vi "GainValue2Number.vi"(10 "GainValue":u64, 11 "Gain permitted values":u32[](array[numeric])=[0, 16, 32, 48, 64, 80, 96, 112, 128, 144, 160, 176, 192, 208, 224, 240, 256, 288, 320, 352, 384, 416, 448, 480, 512, 544, 576, 608, 640, 672, 704, 736, 768, 832, 896, 960, 1024, 1088, 1152, 1216, 1280, 1344, 1408, 1472, 1536, 1600, 1664, 1728]) -> (2 "Value out":u32, 3 "fractional index or x":dbl)   [LabVIEW 2015]
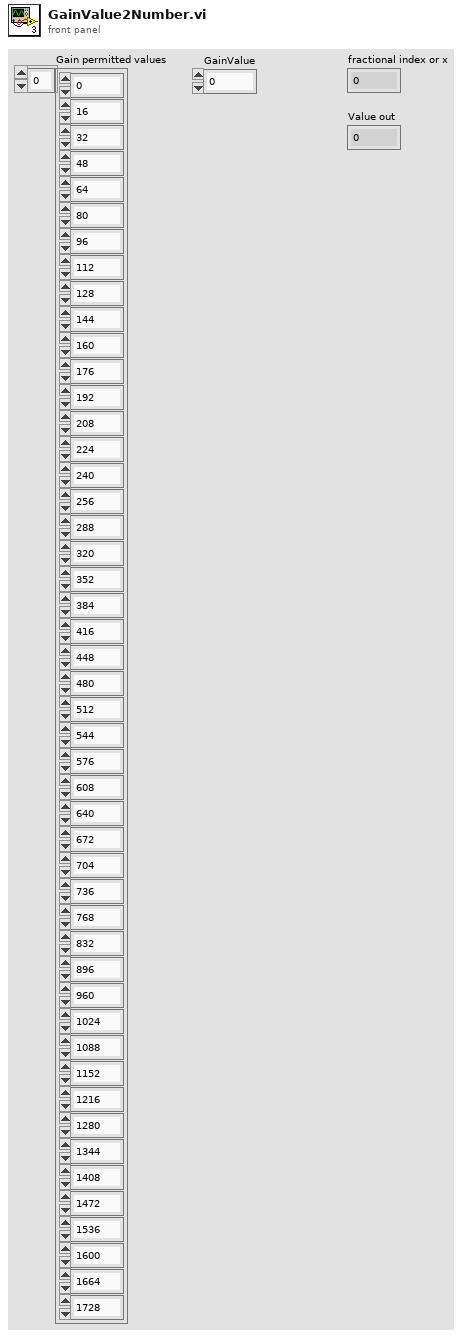
[diagram p1: front panel]
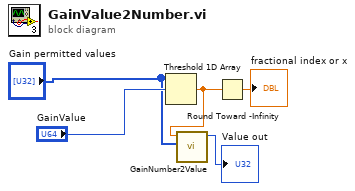
[diagram p0: block diagram]
diagram:
  n1 = Threshold 1D Array(2:"GainValue", 3:"Gain permitted values") -> (0:w2:dbl)  [unwired: 1 in]
  n2 = call "GainNumber2Value.vi"("Gain permitted values"="Gain permitted values", "Numeric"=w2) -> ("Value"=→"Value out":u32)  [unwired: 9 in]
  n3 = Round Toward -Infinity(1:w2) -> (0:→"fractional index or x":dbl)
